vi "Lookup GPIO.vi"(5 "Purpose (None)":string, 7 "Reserve (F)":bool, 8 "error in (no error)":errorcluster, 10 "GPIO #":T1=-1, 11 "Session in":refnum<class "Session.lvclass">) -> (0 "error out":errorcluster, 2 "GPIO":refnum<class "GPIO.lvclass">, 3 "Session out":refnum<class "Session.lvclass">)   [LabVIEW 2020, in "CTI.lvlib" / "Session.lvclass"]
uses:
  Session.lvclass
  Session.lvclass/Session.ctl
  Resource/Resource.lvclass
  GPIO/GPIO.lvclass
  C:/dev/CTI/cti-drivers-lv-visa/CTI/Resource/Resource.lvclass
  C:/dev/CTI/cti-drivers-lv-visa/CTI/GPIO/GPIO.lvclass
  GPIO Number.ctl
  CTI.lvlib
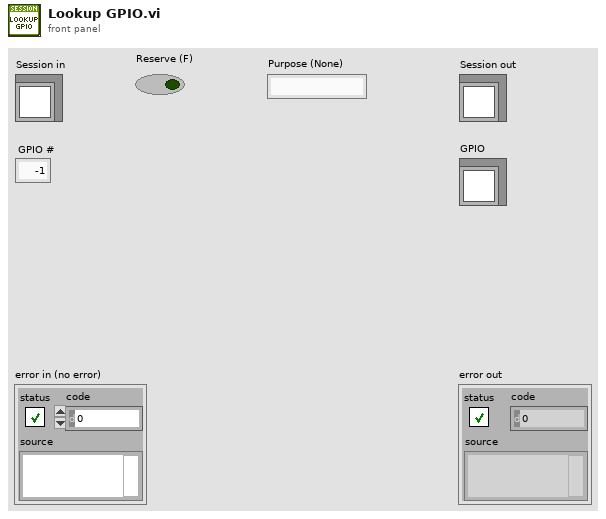
[diagram p1: front panel]
types:
  T1 = typedef "CTI.lvlib/GPIO Number.ctl" = i8
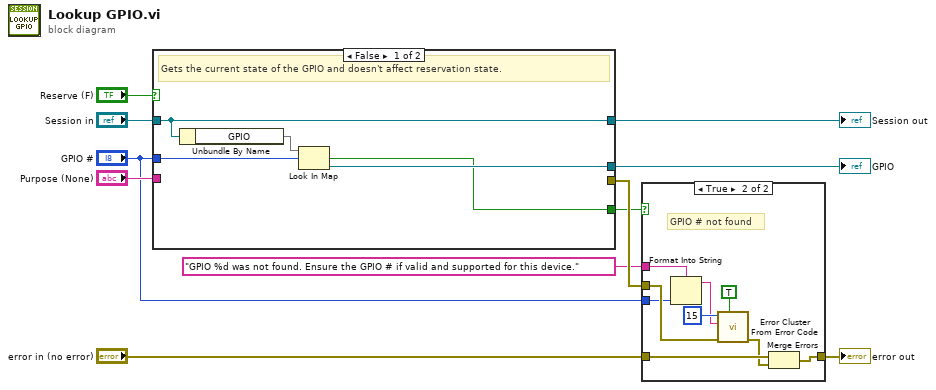
[diagram p0: block diagram]
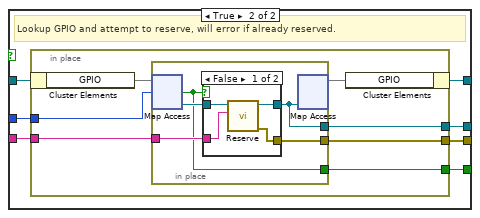
[diagram p2: hidden frame]
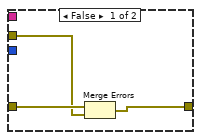
[diagram p4: hidden frame]
diagram:
  n1 = case shown="False" "Reserve (F)" {
    tunnel: "Session in" -> [w12 w23]
    tunnel: "GPIO #" -> [w15 w22]
    tunnel: [w14 w18] -> w8
    tunnel: [w13 w20] -> w5
    tunnel: "Purpose (None)" -> [_ w21]
    tunnel: [w12 w19] -> w6
    tunnel: [_ w17] -> w11
    frame False {
      # "Gets the current state of the GPIO and doesn't affect reservation state."
      n2 = Unbundle By Name(w12) -> ("GPIO"=w16:map{T1, refnum<class "GPIO.lvclass">})
      n3 = Look In Map(map=w16, key=w15) -> (key not found?=w13:bool, value=w14:refnum<class "GPIO.lvclass">)  [unwired: 1 in]
    }
    frame True {
      # "Lookup GPIO and attempt to reserve, will error if already reserved."
      n4 = in-place {
        in-place-border: w22 -> [w29]
        in-place-border: w21 -> [w28]
        in-place-border: [w27] -> w20
        in-place-border: [w25] -> w18
        in-place-border: [w24] -> w17
        n5 = in-place-cluster #1(w23) -> ("GPIO"=w30:map{T1, refnum<class "GPIO.lvclass">})
        n6 = in-place {
          in-place-border: w28 -> [w34]
          in-place-border: [w33] -> w24
          in-place-border: [w32] -> w27
          in-place-border: [w31] -> w25
          n7 = in-place-map #2(w30, w29) -> (w35:refnum<class "GPIO.lvclass">, w32:bool)  [unwired: 1 in]
          n8 = case shown="False" w32 {
            tunnel: w35 -> [w39 w40]
            tunnel: w34 -> [w38 _]
            tunnel: [w37 w40] -> w31
            tunnel: [w36 _] -> w33
            frame False {
              n9 = call "Reserve.vi"("Purpose"=w38, "Resource in"=w39) -> ("error out"=w36:errorcluster, "Resource out"=w37:refnum<class "GPIO.lvclass">)  [unwired: 8 in]
            }
            frame True {
            }
          }
          n10 = in-place-map #2(w31) -> (w26:map{T1, refnum<class "GPIO.lvclass">})  [unwired: 1 in, 2 out]
        }
        n11 = in-place-cluster #1("GPIO"=w26) -> (w19:refnum<class "Session.lvclass">)
      }
    }
  }
  "Session out" <- w6
  "GPIO" <- w8
  n12 = case shown="True" w5 {
    tunnel: w11 -> [w41 w52]
    tunnel: "error in (no error)" -> [w43 w46]
    tunnel: [w42 w44] -> w3
    tunnel: "GPIO %d was not found. Ensure the GPIO # if valid and supported for this device." -> [_ w49]
    tunnel: "GPIO #" -> [_ w48]
    frame False {
      n13 = Merge Errors(w43, w41) -> (w42:errorcluster)
    }
    frame True {
      # "GPIO # not found"
      n14 = Format Into String(format string=w49, w48) -> (resulting string=w47:string)  [unwired: 2 in, 1 out]
      n15 = call <vilib>:"Error Cluster From Error Code.vi"("show call chain? (False)"=TRUE, "error in (no error)"=w52, "error message (\"\")"=w47, "error code (0)"=15) -> ("error out"=w45:errorcluster)  [unwired: 5 in]
      n16 = Merge Errors(w46, w45) -> (w44:errorcluster)
    }
  }
  "error out" <- w3
